vi "plueba2.vi"() -> ()   [LabVIEW 2020]
panel:
  out "imagen decodificada":picture
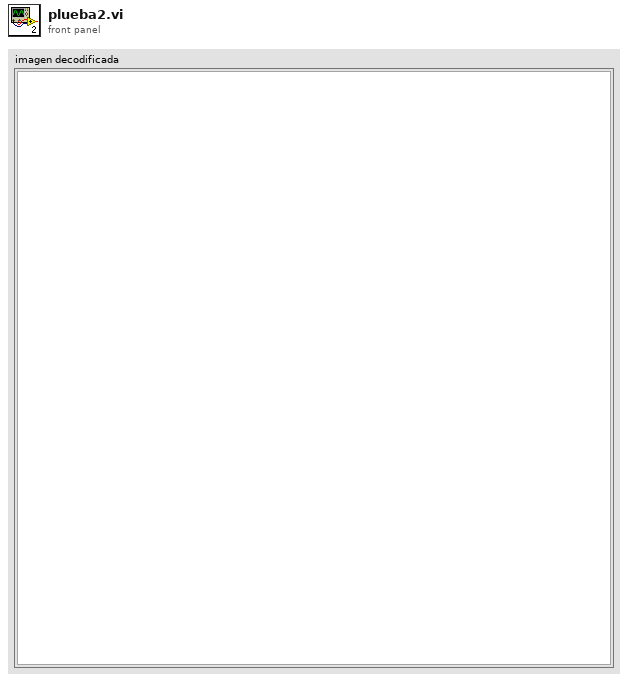
[diagram p1: front panel]
types:
  T1 = enum16{"E1", "E2", "E3", "E4", "E5", "E6", "E7", "E8", "E9"}
  T2 = typedef "imagedata.ctl" = cluster{"image type":i32, "image depth":i32, "image":u8[], "mask":u8[], "colors":u32[], "Rectangle":cluster{"left":i16, "top":i16, "right":i16, "bottom":i16}}
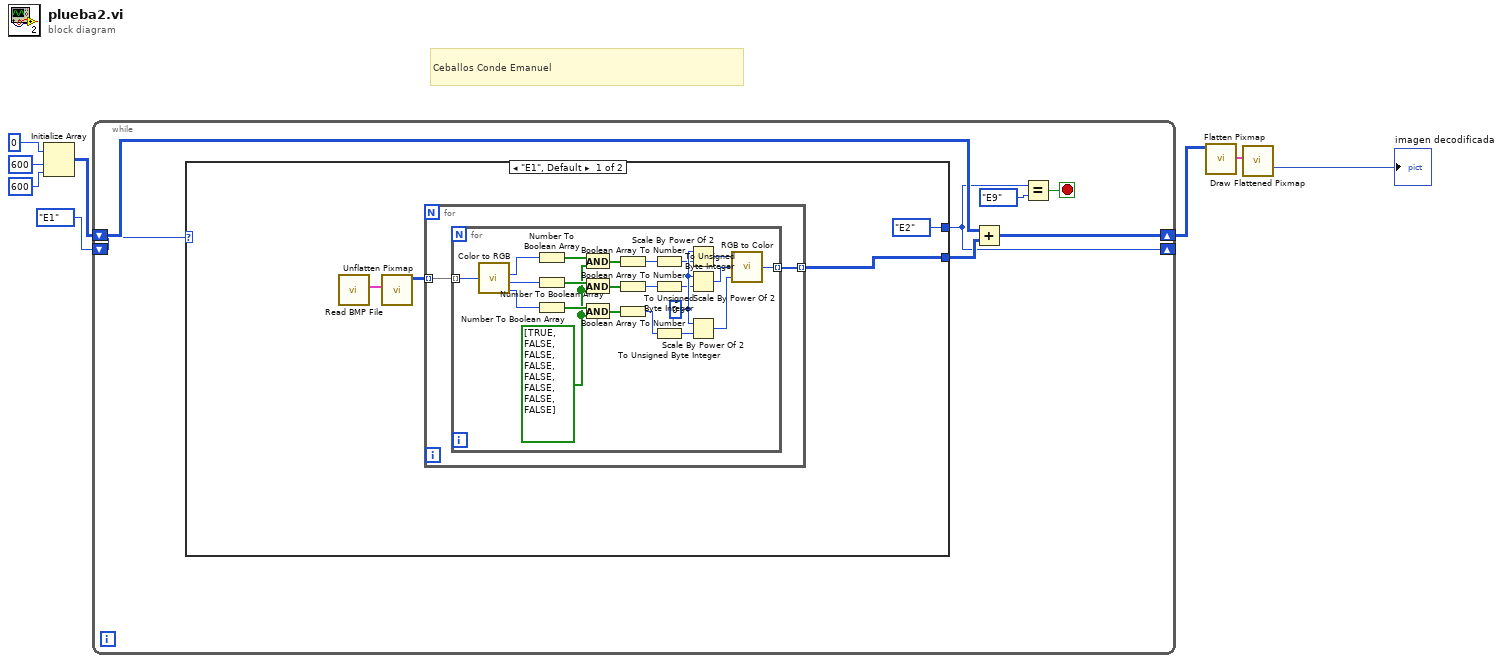
[diagram p0: block diagram]
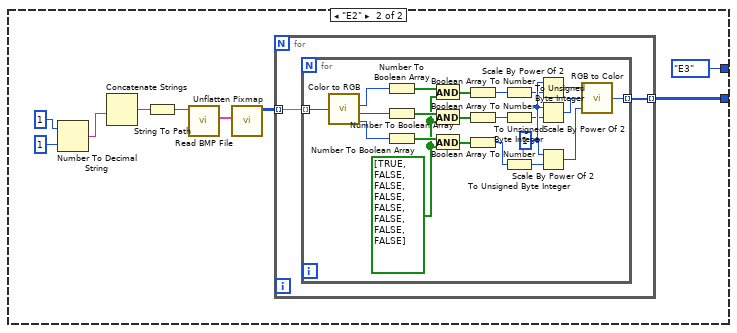
[diagram p2: hidden frame]
diagram:
  # "Ceballos Conde Emanuel"
  n1 = Initialize Array(u32 0 ("element"), 600 ("dimension size"), 600 ("dimension size")) -> (w5:u32[][])
  n2 = while {
    shift-right: [w11] -> _
    shift-left: T1."E1" -> [w9]
    shift-right: [w14] -> w4
    shift-left: w5 -> [w13]
    stop <- w12 stop-if-true
    n3 = case shown="\"E1\", Default" w9 {
      tunnel: [w18 w53] -> w15
      tunnel: [T1."E2" T1."E3"] -> w11
      frame "E1", Default {
        n4 = call <vilib>:"Read BMP File.vi"() -> ("image data"=w17:T2)  [unwired: 9 in, 2 out]
        n5 = call <vilib>:"Unflatten Pixmap.vi"("image data"=w17) -> ("24-bit pixmap"=w19:u32[][])  [unwired: 4 in, 6 out]
        n6 = for {
          tunnel: w19 -> [w21] mode=indexing
          tunnel: [w20] -> w18 mode=indexing
          n7 = for {
            tunnel: w21 -> [w43] mode=indexing
            tunnel: [w26] -> w20 mode=indexing
            w22 = bool[] [TRUE, FALSE, FALSE, FALSE, FALSE, FALSE, FALSE, FALSE] ("Boolean array 7")
            w29 = u8 0 ("x")
            n8 = call <vilib>:"Color to RGB.vi"("Color"=w43) -> ("R"=w40:u8, "G"=w35:u8, "B"=w34:u8)  [unwired: 1 out]
            n9 = Number To Boolean Array(number=w40) -> (Boolean array=w42:bool[])
            n10 = Number To Boolean Array(number=w35) -> (Boolean array=w39:bool[])
            n11 = Number To Boolean Array(number=w34) -> (Boolean array=w37:bool[])
            n12 = And(x=w42, y=w22) -> (x .and. y?=w41:bool[])
            n13 = And(x=w39, y=w22) -> (x .and. y?=w38:bool[])
            n14 = And(x=w37, y=w22) -> (x .and. y?=w36:bool[])
            n15 = Boolean Array To Number(Boolean array=w41) -> (number=w30:u32)
            n16 = Boolean Array To Number(Boolean array=w38) -> (number=w27:u32)
            n17 = Boolean Array To Number(Boolean array=w36) -> (number=w28:u32)
            n18 = To Unsigned Byte Integer(number=w30) -> (unsigned 8bit integer=w25:u8)
            n19 = To Unsigned Byte Integer(number=w27) -> (unsigned 8bit integer=w24:u8)
            n20 = To Unsigned Byte Integer(number=w28) -> (unsigned 8bit integer=w23:u8)
            n21 = Scale By Power Of 2(n=w29, x=w25) -> (x*2^n=w33:u8)
            n22 = Scale By Power Of 2(n=w29, x=w24) -> (x*2^n=w32:u8)
            n23 = Scale By Power Of 2(n=w29, x=w23) -> (x*2^n=w31:u8)
            n24 = call <vilib>:"RGB to Color.vi"("B"=w31, "G"=w32, "R"=w33) -> ("Color"=w26:u32)
          }
        }
      }
      frame "E2" {
        n25 = Number To Decimal String(number=1, width (-)=i16 1) -> (decimal integer string=w45:string)
        n26 = Concatenate Strings(w45) -> (w51:string, w47:string, w46:string, w44:string)
        n27 = String To Path(string=w51) -> (path=w48:path)
        n28 = call <vilib>:"Read BMP File.vi"("path to BMP file"=w48) -> ("image data"=w55:T2)  [unwired: 8 in, 2 out]
        n29 = call <vilib>:"Unflatten Pixmap.vi"("image data"=w55) -> ("24-bit pixmap"=w54:u32[][])  [unwired: 4 in, 6 out]
        n30 = for {
          tunnel: w54 -> [w57] mode=indexing
          tunnel: [w56] -> w53 mode=indexing
          n31 = for {
            tunnel: w57 -> [w79] mode=indexing
            tunnel: [w62] -> w56 mode=indexing
            w58 = bool[] [TRUE, FALSE, FALSE, FALSE, FALSE, FALSE, FALSE, FALSE] ("Boolean array 7")
            w65 = u8 1 ("x")
            n32 = call <vilib>:"Color to RGB.vi"("Color"=w79) -> ("R"=w76:u8, "G"=w71:u8, "B"=w70:u8)  [unwired: 1 out]
            n33 = Number To Boolean Array(number=w76) -> (Boolean array=w78:bool[])
            n34 = Number To Boolean Array(number=w71) -> (Boolean array=w75:bool[])
            n35 = Number To Boolean Array(number=w70) -> (Boolean array=w73:bool[])
            n36 = And(x=w78, y=w58) -> (x .and. y?=w77:bool[])
            n37 = And(x=w75, y=w58) -> (x .and. y?=w74:bool[])
            n38 = And(x=w73, y=w58) -> (x .and. y?=w72:bool[])
            n39 = Boolean Array To Number(Boolean array=w77) -> (number=w66:u32)
            n40 = Boolean Array To Number(Boolean array=w74) -> (number=w63:u32)
            n41 = Boolean Array To Number(Boolean array=w72) -> (number=w64:u32)
            n42 = To Unsigned Byte Integer(number=w66) -> (unsigned 8bit integer=w61:u8)
            n43 = To Unsigned Byte Integer(number=w63) -> (unsigned 8bit integer=w60:u8)
            n44 = To Unsigned Byte Integer(number=w64) -> (unsigned 8bit integer=w59:u8)
            n45 = Scale By Power Of 2(n=w65, x=w61) -> (x*2^n=w69:u8)
            n46 = Scale By Power Of 2(n=w65, x=w60) -> (x*2^n=w68:u8)
            n47 = Scale By Power Of 2(n=w65, x=w59) -> (x*2^n=w67:u8)
            n48 = call <vilib>:"RGB to Color.vi"("B"=w67, "G"=w68, "R"=w69) -> ("Color"=w62:u32)
          }
        }
      }
    }
    n49 = Add(x=w13, y=w15) -> (x+y=w14:u32[][])
    n50 = Equal?(x=w11, y=T1."E9") -> (x = y?=w12:bool)
  }
  n51 = call <vilib>:"Flatten Pixmap.vi"("24-bit pixmap"=w4) -> ("image data"=w2:T2)  [unwired: 10 in]
  n52 = call <vilib>:"Draw Flattened Pixmap.vi"("image data"=w2) -> ("new picture"=→"imagen decodificada":picture)  [unwired: 8 in]
